vi "Tank Arcade Control.vi"(6 "Max Output":dbl=1.0, 7 "Square Inputs":bool=TRUE, 9 "Y axis value":dbl, 10 "X axis value":dbl) -> (1 "Right Motor Value":dbl, 2 "Left Motor Value":dbl)   [LabVIEW 2015]
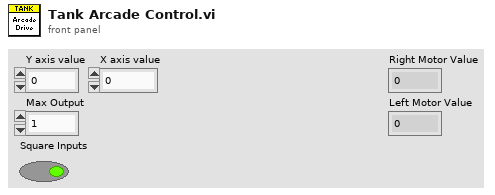
[diagram p1: front panel]
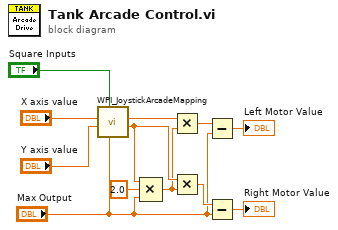
[diagram p0: block diagram]
diagram:
  n1 = call <vilib>:"WPI_JoystickArcadeMapping.vi"("Max Output"="Max Output", "Square Inputs"="Square Inputs", "Y axis value"="Y axis value", "X axis value"="X axis value") -> ("Right Motor Value"=w4:dbl, "Left Motor Value"=w9:dbl)  [unwired: 6 in]
  n2 = Compound Arithmetic op=MULTIPLY(w4, 2.0 ("y"), "Max Output") -> (w2:dbl)
  n3 = Multiply(x=w9, y=w2) -> (x*y=w5:dbl)
  n4 = Multiply(x=w4, y=w2) -> (x*y=w6:dbl)
  n5 = Subtract(x=w5, y="Max Output") -> (x-y=→"Left Motor Value":dbl)
  n6 = Subtract(x=w6, y="Max Output") -> (x-y=→"Right Motor Value":dbl)
